vi "Configure Occupied Bandwidth.vi"(0 "VISA resource name":refnum<visa-resource-name>, 5 "OBW Method (0:N%)":i32(ring) items=["N%", "XdB"], 7 "OBW Ratio (99.00%)":dbl=99.0 min=0.01 max=99.99 format="%.2f", 9 "OBW Level (20.00dB)":dbl=20.0 min=0.01 max=100.0 format="%.2f", 11 "error in (no error)":errorcluster) -> (4 "VISA resource name out":refnum<visa-resource-name>, 15 "error out":errorcluster)   [LabVIEW 2020, in "Anritsu Signal Analyzer Series.lvlib"]
doc: "Configures the Occupied Bandwidth settings of the spectrum analyzer."
uses:
  Anritsu Signal Analyzer Series.lvlib
panel:
  # "%"
  # "dB"
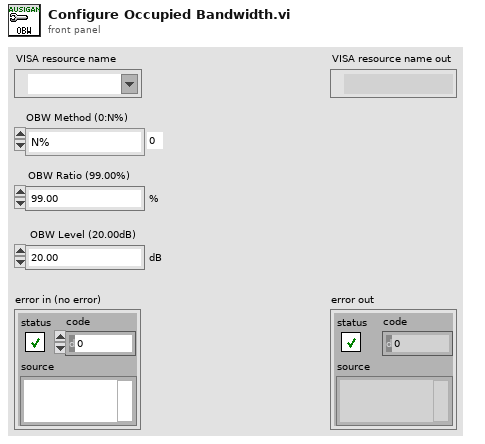
[diagram p1: front panel]
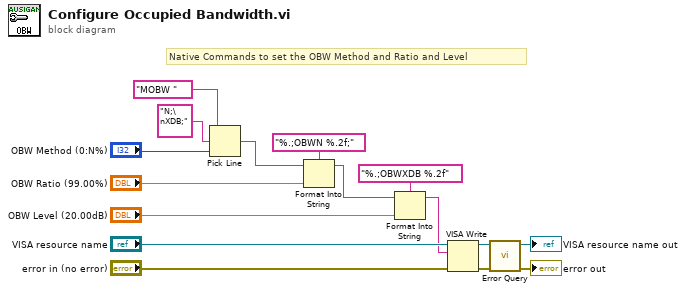
[diagram p0: block diagram]
diagram:
  # "Native Commands to set the OBW Method and Ratio and Level"
  n1 = Pick Line(string ("")="MOBW " ("_CommandSet"), multi-line string="N;\nXDB;" ("複数行文字列"), line index="OBW Method (0:N%)") -> (output string=w3:string)
  n2 = Format Into String(format string="%.;OBWN %.2f;" ("Format String"), initial string=w3, "OBW Ratio (99.00%)") -> (resulting string=w6:string)  [unwired: 1 in, 1 out]
  n3 = Format Into String(format string="%.;OBWXDB %.2f" ("Format String"), initial string=w6, "OBW Level (20.00dB)") -> (resulting string=w5:string)  [unwired: 1 in, 1 out]
  n4 = VISA Write(VISA resource name="VISA resource name", write buffer=w5, error in (no error)="error in (no error)") -> (VISA resource name out=w10:refnum<visa-resource-name>, error out=w9:errorcluster)  [unwired: 1 out]
  n5 = call "Error Query.vi"("error in (no error)"=w9, "VISA resource name"=w10) -> ("error out"=→"error out":errorcluster, "VISA resource name out"=→"VISA resource name out":refnum<visa-resource-name>)  [unwired: 6 in, 2 out]
